vi "Initialize AO Channels.vi"(8 "error in (no error)":errorcluster, 11 "Instrument.Lockin in":refnum<class "Instrument.Lockin.lvclass">) -> (0 "error out":errorcluster, 3 "Instrument.Lockin out":refnum<class "Instrument.Lockin.lvclass">)   [LabVIEW 2016, in "Instrument.Lockin.lvclass"]
uses:
  Instrument.Lockin.lvclass
  Instrument.Lockin.lvclass/Instrument.Lockin.ctl
  Typedefs/Function-enum.ctl
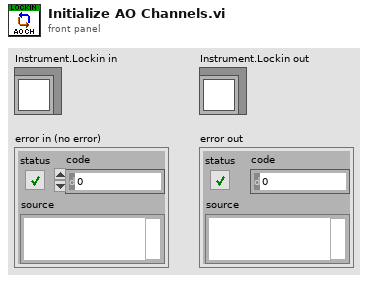
[diagram p1: front panel]
types:
  T1 = typedef "Instrument.Lockin.lvclass/AO-cluster.ctl" = cluster{"AO Amp (V)":T2, "AO DC (V)":T3, "AO f (Hz)":T4, "AO Phase (°)":T5, "Function":T6, "I+":bool[], "Sweeping":bool[]}
  T2 = typedef "Instrument.Lockin.lvclass/AO_Amp-array.ctl" = dbl[]
  T3 = typedef "Instrument.Lockin.lvclass/AO_DC-array.ctl" = dbl[]
  T4 = typedef "Instrument.Lockin.lvclass/AO_f-array.ctl" = dbl[]
  T5 = typedef "Instrument.Lockin.lvclass/AO_phi-array.ctl" = dbl[]
  T6 = typedef "Instrument.Lockin.lvclass/Function-array.ctl" = T7[]
  T7 = typedef "Instrument.Lockin.lvclass/Function-enum.ctl" = enum16{"Sine", "Triangle", "Square", "Sawtooth"}
  T8 = typedef "Instrument.Lockin.lvclass/AO.config-array.ctl" = T9[]
  T9 = typedef "Instrument.Lockin.lvclass/AO.config-cluster.ctl" = cluster{"AO.channels":tag, "AO.Range":T10, "output terminal configuration":i32, "DAQ Type":T11}
  T10 = typedef "Instrument.Lockin.lvclass/446xAO-enum.ctl" = enum16{"±0.1 V", "±1.0 V", "±10.0 V"}
  T11 = typedef "Instrument.Lockin.lvclass/DAQType-enum.ctl" = enum16{"None", "USB 4431", "PXI 446x"}
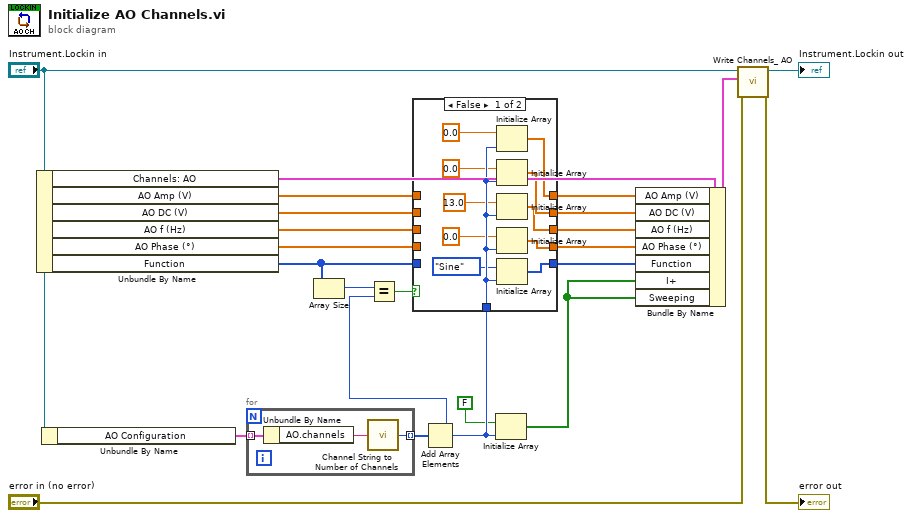
[diagram p0: block diagram]
diagram:
  n1 = Unbundle By Name("Instrument.Lockin in") -> ("Channels: AO"=w21:T1, "AO Amp (V)"=w16:T2, "AO DC (V)"=w17:T3, "AO f (Hz)"=w18:T4, "AO Phase (°)"=w19:T5, "Function"=w20:T6)
  n2 = Unbundle By Name("Instrument.Lockin in") -> ("AO Configuration"=w15:T8)
  n3 = for {
    tunnel: w15 -> [w26] mode=indexing
    tunnel: [w24] -> w4 mode=indexing
    n4 = Unbundle By Name(w26) -> ("AO.channels"=w25:tag)
    n5 = call "Channel String to Number of Channels.vi"("Channels String"=w25) -> ("# channels"=w24:i32)  [unwired: 4 in]
  }
  n6 = Array Size(array=w20) -> (size(s)=w6:i32)
  n7 = Add Array Elements(numeric array=w4) -> (sum=w14:i32)
  n8 = Equal?(x=w6, y=w14) -> (x = y?=w8:bool)
  n9 = case shown="False" w8 {
    tunnel: [w35 w42] -> w9
    tunnel: w20 -> [_ w42]
    tunnel: [w34 w38] -> w10
    tunnel: [w32 w41] -> w11
    tunnel: w18 -> [_ w41]
    tunnel: [w33 w40] -> w12
    tunnel: w17 -> [_ w40]
    tunnel: [w36 w39] -> w13
    tunnel: w16 -> [_ w39]
    tunnel: w14 -> [w37 _]
    tunnel: w19 -> [_ w38]
    frame False {
      n10 = Initialize Array(0.0, w37) -> (w36:dbl[])
      n11 = Initialize Array(0.0, w37) -> (w33:dbl[])
      n12 = Initialize Array(13.0, w37) -> (w32:dbl[])
      n13 = Initialize Array(0.0, w37) -> (w34:dbl[])
      n14 = Initialize Array(Function-enum."Sine" ("Signal Type"), w37) -> (w35:T7[])
    }
    frame True {
    }
  }
  n15 = Initialize Array(FALSE, w14) -> (w7:bool[])
  n16 = Bundle By Name(cluster=w21, "AO Amp (V)"=w13, "AO DC (V)"=w12, "AO f (Hz)"=w11, "AO Phase (°)"=w10, "Function"=w9, "I+"=w7, "Sweeping"=w7) -> (w22:T1)
  n17 = call "Write Channels_ AO.vi"("error in (no error)"="error in (no error)", "Channels: AO"=w22, "Instrument.Lockin in"="Instrument.Lockin in") -> ("error out"=→"error out":errorcluster, "Instrument.Lockin out"=→"Instrument.Lockin out":refnum<class "Instrument.Lockin.lvclass">)  [unwired: 7 in]
